vi "Update PV.vi"(8 "error in (no error)":errorcluster, 10 "PV":refnum<class "PV.lvclass">, 11 "CS++ScopeGui in":refnum<class "CS++ScopeGui.lvclass">) -> (0 "error out":errorcluster, 3 "CS++ScopeGui out":refnum<class "CS++ScopeGui.lvclass">)   [LabVIEW 2013, in "CS++ScopeGui.lvlib" / "CS++ScopeGui.lvclass"]
uses:
  CS++ScopeGui.lvclass
  CSPP_Core/Classes/CS++ProcessVariables/ProcessVariable/PV.lvclass
  CS++ScopeGui.lvclass/CS++ScopeGui.ctl
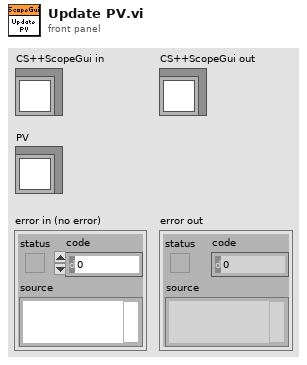
[diagram p1: front panel]
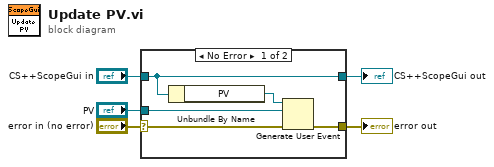
[diagram p0: block diagram]
diagram:
  n1 = case shown="No Error" "error in (no error)" {
    selector: "error in (no error)" -> [w10 w12]
    tunnel: [w9 w12] -> w4
    tunnel: [w8 w11] -> w2
    tunnel: "CS++ScopeGui in" -> [w8 w11]
    tunnel: "PV" -> [w6 _]
    frame No Error {
      n2 = Unbundle By Name(w8) -> ("PV"=w7:refnum<user-event>)
      n3 = Generate User Event(user event=w7, event data cluster=w6, error in=w10) -> (error out=w9:errorcluster)  [unwired: 1 in, 1 out]
    }
    frame Error {
    }
  }
  "error out" <- w4
  "CS++ScopeGui out" <- w2
